vi "thcd_set_ahy.vi"(5 "thcd_delay":u32=500, 6 "err_in":errorcluster, 7 "thcd_val":i32 min=0 max=250 step=1, 8 "thcd_ch":T1, 9 "thcd_visa":refnum<visa-resource-name>) -> (0 "err_out":errorcluster, 1 "thcd_st":bool, 2 "thcd_res_msg":string, 3 "thcd_visa":refnum<visa-resource-name>)   [LabVIEW 2019]
uses:
  thcd_controls/ctrl_chn_thcd.ctl
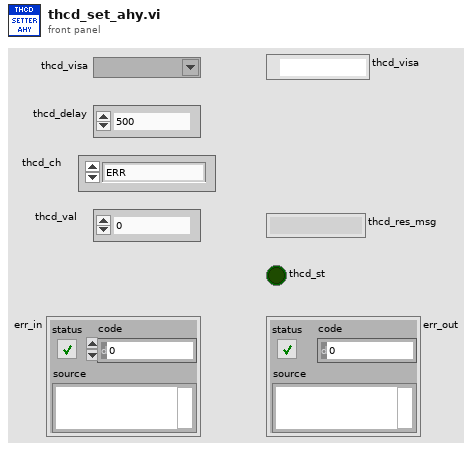
[diagram p1: front panel]
types:
  T1 = typedef "ctrl_chn_thcd.ctl" = enum8{"ERR", "1", "2", "3", "4"}
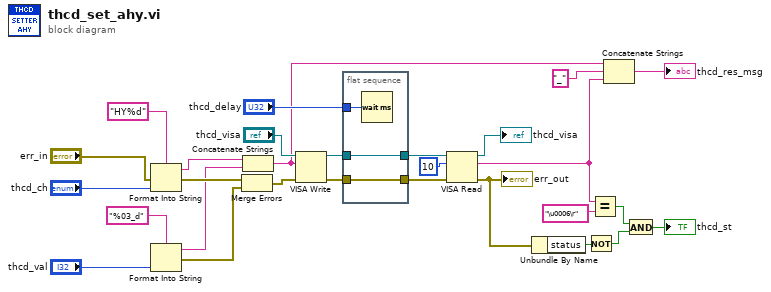
[diagram p0: block diagram]
diagram:
  n1 = Format Into String(format string="HY%d", error in="err_in", "thcd_ch") -> (resulting string=w20:string, error out=w19:errorcluster)  [unwired: 1 in]
  n2 = Format Into String(format string="%03_d", "thcd_val") -> (resulting string=w16:string, error out=w17:errorcluster)  [unwired: 2 in]
  n3 = Merge Errors(w19, w17) -> (w18:errorcluster)
  n4 = Concatenate Strings(w20, w16) -> (w3:string)
  n5 = VISA Write(VISA resource name="thcd_visa", write buffer=w3, error in (no error)=w18) -> (VISA resource name out=w27:refnum<visa-resource-name>, error out=w28:errorcluster)  [unwired: 1 out]
  n6 = flat-sequence {
    tunnel: w28 -> [w30]
    tunnel: [w30] -> w7
    tunnel: w27 -> [w29]
    tunnel: [w29] -> w6
    tunnel: "thcd_delay" -> [w31]
    frame #0 {
      n7 = Wait (ms)(milliseconds to wait=w31) -> ()  [unwired: 1 out]
    }
  }
  n8 = VISA Read(VISA resource name=w6, byte count=u32 10, error in (no error)=w7) -> (VISA resource name out=→"thcd_visa":refnum<visa-resource-name>, read buffer=w8:string, error out=w4:errorcluster)  [unwired: 1 out]
  "err_out" <- w4
  n9 = Unbundle By Name(w4) -> ("status"=w14:bool)
  n10 = Not(x=w14) -> (.not. x?=w11:bool)
  n11 = Equal?(x=w8, y="\u0006\r") -> (x = y?=w12:bool)
  n12 = Concatenate Strings(w3, "_", w8) -> (→"thcd_res_msg":string)
  n13 = And(x=w12, y=w11) -> (x .and. y?=→"thcd_st":bool)
